vi "_Parse SEM Segment Margin Result.vi"(8 "error in (no error)":errorcluster, 10 "Input String":string, 11 "VISA resource name":refnum<visa-resource-name>) -> (0 "error out":errorcluster, 1 "SEM Offset Results":cluster{"Margin X":dbl, "Margin Y":dbl}[](array[cluster]) {"Margin Y" format="%^.3e"; "Margin X" format="%^.3e"}, 2 "Reliability Results":T1, 3 "VISA resource name out":refnum<visa-resource-name>, 5 "Out Of Tolerance":dbl format="%^.3e", 7 "Statistic Expired":i32)   [LabVIEW 2015, in "Rohde&Schwarz CMXP NR FR2 Measurement.lvlib"]
uses:
  <instrlib>/Rohde&Schwarz CMXP NR FR2 Measurement/Rohde&Schwarz CMXP NR FR2 Measurement.lvlib
  <instrlib>/Rohde&Schwarz CMXP NR FR2 Measurement/Private/rsidr_core.llb/rsidr_core.lvlib
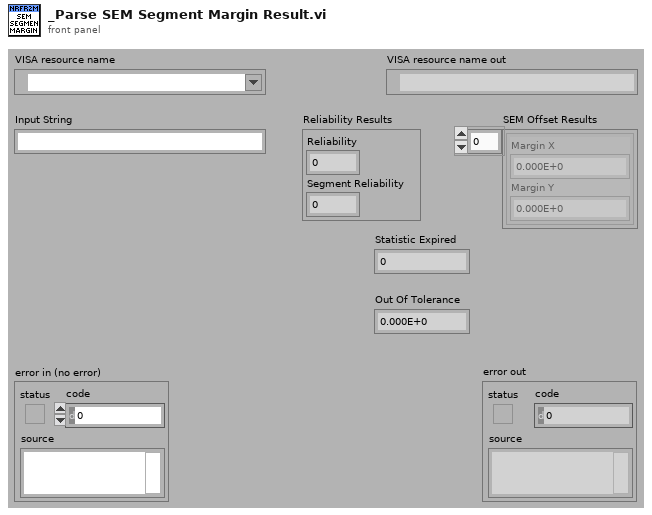
[diagram p1: front panel]
types:
  T1 = cluster{"Reliability":i32, "Segment Reliability":i32}
  T2 = cluster{"double array out[0]":dbl, "double array out[1]":dbl}
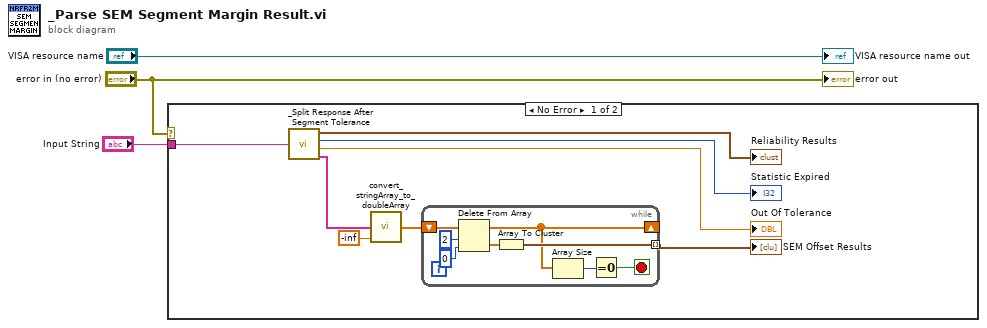
[diagram p0: block diagram]
diagram:
  n1 = case shown="No Error" "error in (no error)" {
    tunnel: "Input String" -> [w4 _]
    frame No Error {
      n2 = call <instrlib>:"_Split Response After Segment Tolerance.vi"("Input String"=w4) -> ("Reliability Results"=→"Reliability Results":T1, "Statistic Expired"=→"Statistic Expired":i32, "Out Of Tolerance"=→"Out Of Tolerance":dbl, "Response out"=w11:string[])
      n3 = call <instrlib>:"convert_stringArray_to_doubleArray.vi"("default (0)"=-inf, "string array in"=w11) -> ("double array out"=w6:dbl[])  [unwired: 3 in]
      n4 = while {
        shift-right: [w14] -> _
        shift-left: w6 -> [w19]
        tunnel: [w15] -> w5 mode=indexing
        stop <- w12 stop-if-true
        n5 = Delete From Array(array=w19, length=2, index=0) -> (deleted portion=w16:dbl[], array with subset deleted=w14:dbl[])
        n6 = Array To Cluster(array=w16) -> (cluster=w15:T2)
        n7 = Array Size(array=w14) -> (size(s)=w13:i32)
        n8 = Equal To 0?(x=w13) -> (x = 0?=w12:bool)
      }
      "SEM Offset Results" <- w5
    }
    frame Error {
    }
  }
  "error out" <- "error in (no error)"
  "VISA resource name out" <- "VISA resource name"
